vi "Get child hwnd.vi"(8 "Error In":errorcluster, 11 "MDI.lvlib:Document.lvclass":refnum<class "Document.lvclass">) -> (0 "Error Out":errorcluster, 2 "Child hWnd":u32, 3 "MDI.lvlib:Document.lvclass 2":refnum<class "Document.lvclass">)   [LabVIEW 2016, in "Document.lvclass"]
uses:
  Document.lvclass
  Document.lvclass/Document.ctl
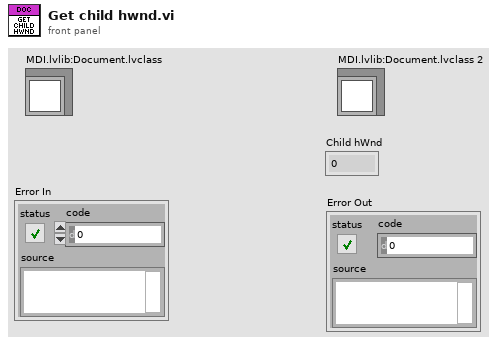
[diagram p1: front panel]
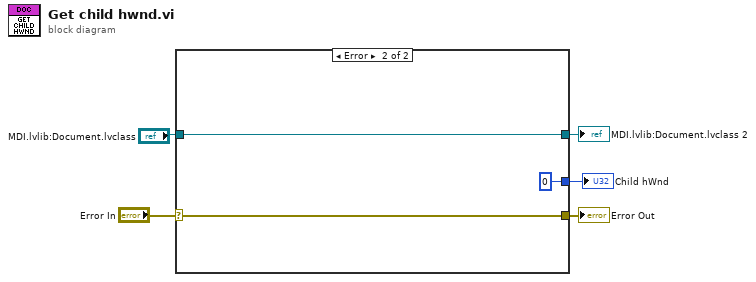
[diagram p0: block diagram]
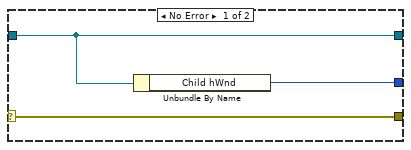
[diagram p2: hidden frame]
diagram:
  n1 = case shown="Error" "Error In" {
    selector: "Error In" -> [w8 w11]
    tunnel: [w8 w11] -> w4
    tunnel: [w7 u32 0 ("Child hWnd")] -> w3
    tunnel: "MDI.lvlib:Document.lvclass" -> [w6 w9]
    tunnel: [w6 w9] -> w1
    frame No Error {
      n2 = Unbundle By Name(w6) -> ("Child hWnd"=w7:u32)
    }
    frame Error {
    }
  }
  "Error Out" <- w4
  "Child hWnd" <- w3
  "MDI.lvlib:Document.lvclass 2" <- w1
